vi "Benchmark Build Table.vi"() -> ()   [LabVIEW 2017]
uses:
  Source/LookupTable/LookupTable.lvclass/LookupTable.ctl
  694ccc22-8164-4270-828e-5d368f579845.vi
  Source/LookupTable/Read Table Reference.vi
  Source/LookupTable/LookupTable.lvclass
panel:
  in  "Table Size":i32=100000
  out "Waveform Chart":cluster{dbl, dbl, dbl}(graph)
  out "Variant by Reference":dbl
  out "Variant by value":dbl
  out "Composed Lookup Table":dbl
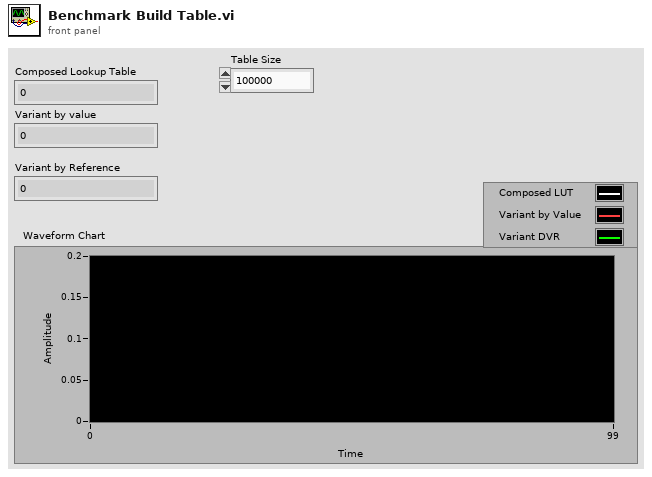
[diagram p1: front panel]
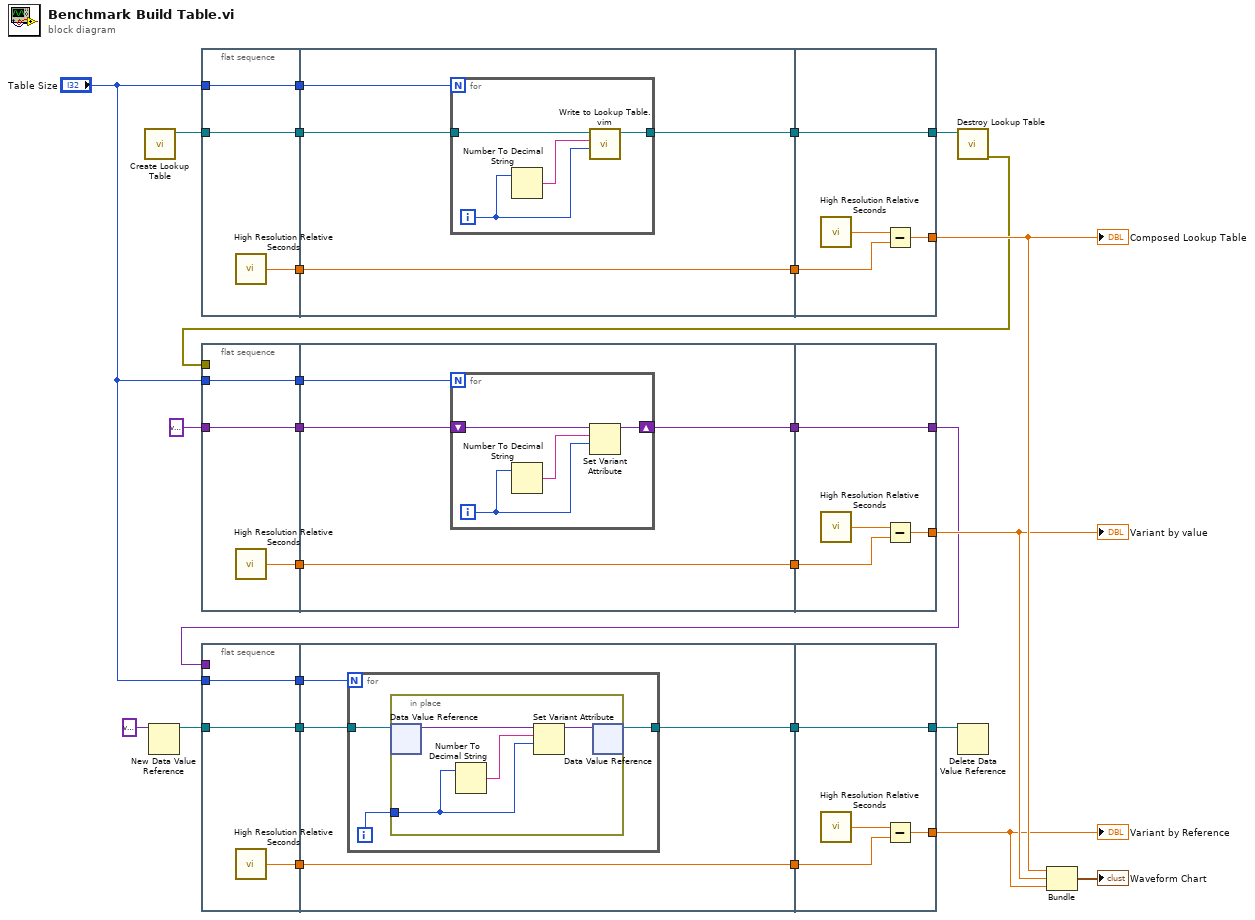
[diagram p0: block diagram]
diagram:
  n1 = call "Create Lookup Table.vi"() -> ("LookupTable Reference"=w23:refnum<data-value>)  [unwired: 10 in, 1 out]
  n2 = New Data Value Reference(data value=variant) -> (data value reference=w12:refnum<data-value>)  [unwired: 1 in, 1 out]
  n3 = flat-sequence {
    tunnel: [w31] -> w28
    tunnel: [w30] -> w24
    tunnel: w23 -> [w30]
    tunnel: [w29] -> w20
    tunnel: "Table Size" -> [w29]
    tunnel: w28 -> [w35]
    tunnel: [w35] -> w27
    tunnel: w24 -> [w32]
    tunnel: [w34] -> w21
    tunnel: w20 -> [w33]
    tunnel: w27 -> [w42]
    tunnel: [w41] -> w9
    tunnel: [w40] -> w22
    tunnel: w21 -> [w40]
    frame #0 {
      n4 = call <vilib>:"High Resolution Relative Seconds.vi"() -> ("relative seconds"=w31:dbl)
    }
    frame #1 {
      n5 = for {
        N: w33 -> [_]
        tunnel: [w37] -> w34
        tunnel: w32 -> [w36]
        i -> [w38]
        n6 = Number To Decimal String(number=w38) -> (decimal integer string=w39:string)  [unwired: 1 in]
        n7 = call "Write to Lookup Table.vim"("Item"=w38, "Item Name"=w39, "LookupTable Reference"=w36) -> ("LookupTable Reference Out"=w37:refnum<data-value>)  [unwired: 6 in, 2 out]
      }
    }
    frame #2 {
      n8 = call <vilib>:"High Resolution Relative Seconds.vi"() -> ("relative seconds"=w43:dbl)
      n9 = Subtract(x=w43, y=w42) -> (x-y=w41:dbl)
    }
  }
  n10 = flat-sequence {
    tunnel: [w46] -> w26
    tunnel: [w45] -> w19
    tunnel: "Table Size" -> [w45]
    tunnel: [w44] -> w5
    tunnel: variant -> [w44]
    tunnel: w2 -> [_]
    tunnel: w26 -> [w50]
    tunnel: [w50] -> w25
    tunnel: w19 -> [w49]
    tunnel: w5 -> [w48]
    tunnel: [w47] -> w3
    tunnel: w25 -> [w57]
    tunnel: [w56] -> w8
    tunnel: [w55] -> w1
    tunnel: w3 -> [w55]
    frame #0 {
      n11 = call <vilib>:"High Resolution Relative Seconds.vi"() -> ("relative seconds"=w46:dbl)
    }
    frame #1 {
      n12 = for {
        N: w49 -> [_]
        shift-right: [w54] -> w47
        shift-left: w48 -> [w51]
        i -> [w52]
        n13 = Number To Decimal String(number=w52) -> (decimal integer string=w53:string)  [unwired: 1 in]
        n14 = Set Variant Attribute(Variant=w51, name=w53, value=w52) -> (Variant out=w54:variant)  [unwired: 1 in, 2 out]
      }
    }
    frame #2 {
      n15 = call <vilib>:"High Resolution Relative Seconds.vi"() -> ("relative seconds"=w58:dbl)
      n16 = Subtract(x=w58, y=w57) -> (x-y=w56:dbl)
    }
  }
  n17 = flat-sequence {
    tunnel: [w61] -> w18
    tunnel: [w60] -> w17
    tunnel: "Table Size" -> [w60]
    tunnel: [w59] -> w13
    tunnel: w12 -> [w59]
    tunnel: w1 -> [_]
    tunnel: w18 -> [w65]
    tunnel: [w65] -> w16
    tunnel: w17 -> [w64]
    tunnel: w13 -> [w63]
    tunnel: [w62] -> w11
    tunnel: w16 -> [w75]
    tunnel: [w74] -> w7
    tunnel: [w73] -> w10
    tunnel: w11 -> [w73]
    frame #0 {
      n18 = call <vilib>:"High Resolution Relative Seconds.vi"() -> ("relative seconds"=w61:dbl)
    }
    frame #1 {
      n19 = for {
        N: w64 -> [_]
        tunnel: w63 -> [w68]
        tunnel: [w66] -> w62
        i -> [w67]
        n20 = in-place {
          in-place-border: w67 -> [w69]
          n21 = in-place-dvr #1(w68) -> (w71:variant)  [unwired: 1 out]
          n22 = Number To Decimal String(number=w69) -> (decimal integer string=w72:string)  [unwired: 1 in]
          n23 = Set Variant Attribute(Variant=w71, name=w72, value=w69) -> (Variant out=w70:variant)  [unwired: 1 in, 2 out]
          n24 = in-place-dvr #1(w70) -> (w66:refnum<data-value>)  [unwired: 1 out]
        }
      }
    }
    frame #2 {
      n25 = call <vilib>:"High Resolution Relative Seconds.vi"() -> ("relative seconds"=w76:dbl)
      n26 = Subtract(x=w76, y=w75) -> (x-y=w74:dbl)
    }
  }
  n27 = call "Destroy Lookup Table.vi"("LookupTable Reference"=w22) -> ("error out"=w2:errorcluster)  [unwired: 10 in]
  n28 = Delete Data Value Reference(data value reference=w10) -> ()  [unwired: 1 in, 2 out]
  n29 = Bundle(w9, w8, w7) -> (→"Waveform Chart":cluster{dbl, dbl, dbl})  [unwired: 1 in]
  "Composed Lookup Table" <- w9
  "Variant by value" <- w8
  "Variant by Reference" <- w7
